vi "New Malleable VI.vi"(8 "error in (no error)":errorcluster, 10 "App Refnum":refnum<vi>, 11 "SubVI Refnum":refnum<vi>) -> (0 "error out":errorcluster, 3 "Malleable VI Type out":refnum<class "Malleable VI Type.lvclass">)   [LabVIEW 2020, in "Peek Window.lvlib" / "Malleable VI Type.lvclass"]
uses:
  Malleable VI Type.lvclass
  D:/Code/VI-Peek/source/Peek Window/VI Types/Standard VI Type/Standard VI Type.lvclass
  Implementation VI Type/Implementation VI Type.lvclass
  Selected Implementation Enum.ctl
  Standard VI Type/Standard VI Type.lvclass/Standard VI Type.ctl
  Malleable VI Type.lvclass/Malleable VI Type.ctl
  Standard VI Type/Write VI Refnum.vi
  Standard VI Type/Write App Refnum.vi
  Standard VI Type/Write Full Qualified Name.vi
  Standard VI Type/Write Openable.vi
  Standard VI Type/Write Selectable.vi
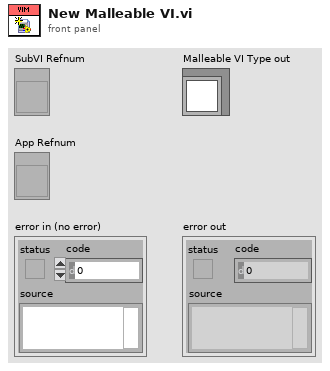
[diagram p1: front panel]
types:
  T1 = typedef "Peek Window.lvlib/Malleable VI Type.lvclass/Selected Implementation Enum.ctl" = enum16{"Actual", "Instance"}
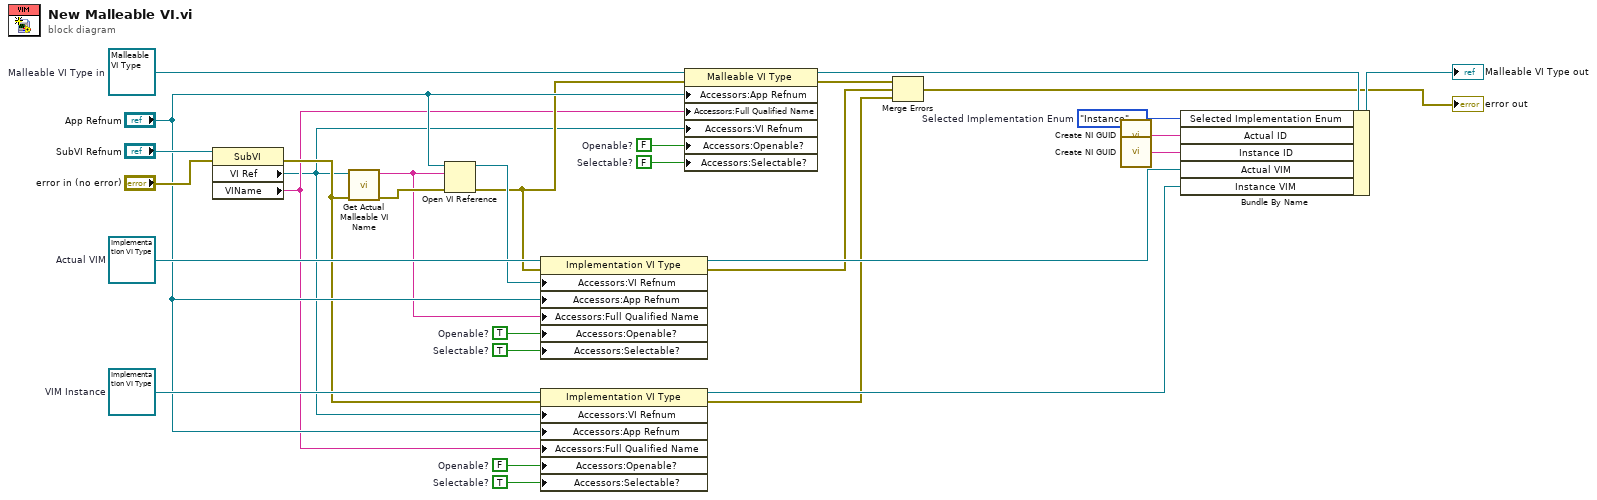
[diagram p0: block diagram]
diagram:
  w13 = TRUE  # Selectable?
  w15 = FALSE  # Openable?
  w16 = TRUE  # Selectable?
  w17 = TRUE  # Openable?
  w18 = FALSE  # Selectable?
  w19 = FALSE  # Openable?
  w22 = refnum<class "Implementation VI Type.lvclass"> refnum  # Actual VIM
  w24 = Selected_Implementation_Enum."Instance"  # Selected Implementation Enum
  w30 = refnum<class "Implementation VI Type.lvclass"> refnum  # VIM Instance
  w28 = refnum<class "Malleable VI Type.lvclass"> refnum  # Malleable VI Type in
  n1 = property class="SubVI"(reference="SubVI Refnum", error in="error in (no error)") -> (error out=w20:errorcluster, "VI Ref"=w1:refnum<vi>, "VIName"=w3:string)  [unwired: 1 out]
  n2 = call "Get Actual Malleable VI Name.vi"("error in"=w20, "VI Reference"=w1) -> ("error out"=w5:errorcluster, "Malleable VI Full Qualified Name"=w2:string)  [unwired: 8 in]
  n3 = Open VI Reference(application reference (local)="App Refnum", vi path=w2, error in (no error)=w5) -> (vi reference=w14:refnum<vi>, error out=w4:errorcluster)  [unwired: 3 in]
  n4 = property class="Implementation VI Type"(reference=w22, error in=w4, "Accessors:VI Refnum"=w14, "Accessors:App Refnum"="App Refnum", "Accessors:Full Qualified Name"=w2, "Accessors:Openable?"=w17, "Accessors:Selectable?"=w16) -> (reference out=w10:refnum<class "Implementation VI Type.lvclass">, error out=w7:errorcluster)
  n5 = property class="Implementation VI Type"(reference=w30, error in=w20, "Accessors:VI Refnum"=w1, "Accessors:App Refnum"="App Refnum", "Accessors:Full Qualified Name"=w3, "Accessors:Openable?"=w15, "Accessors:Selectable?"=w13) -> (reference out=w9:refnum<class "Implementation VI Type.lvclass">, error out=w6:errorcluster)
  n6 = property class="Malleable VI Type"(reference=w28, error in=w4, "Accessors:App Refnum"="App Refnum", "Accessors:Full Qualified Name"=w3, "Accessors:VI Refnum"=w1, "Accessors:Openable?"=w19, "Accessors:Selectable?"=w18) -> (reference out=w23:refnum<class "Malleable VI Type.lvclass">, error out=w26:errorcluster)
  n7 = Merge Errors(w26, w7, w6) -> (→"error out":errorcluster)
  n8 = call <vilib>:"Create NI GUID.vi"() -> ("NI GUID"=w12:string)
  n9 = call <vilib>:"Create NI GUID.vi"() -> ("NI GUID"=w11:string)
  n10 = Bundle By Name(cluster=w23, "Selected Implementation Enum"=w24, "Actual ID"=w12, "Instance ID"=w11, "Actual VIM"=w10, "Instance VIM"=w9) -> (→"Malleable VI Type out":refnum<class "Malleable VI Type.lvclass">)
